vi "_MISC_ Cursor2Center.vi"(8 "Error In":errorcluster, 11 "WaveformGraph Ref":refnum<vi>) -> (0 "Error Out":errorcluster, 3 "XY":cluster{"X":dbl, "Y":dbl})   [LabVIEW 2014]
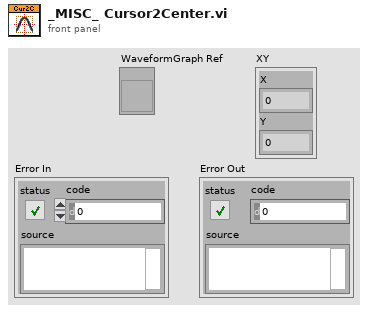
[diagram p1: front panel]
types:
  T1 = typedef "LVCursorListTypeDef.ctl" = cluster{"Name":string, "Color":u32, "Style":u8, "Point Style":u8, "Name Visible":bool, "Allow Drag":bool, "Cursor Mode":u32, "Plot":i32, "Index":i32, "Position":cluster{"X":dbl, "Y":dbl}, "X Scale":u32, "Y Scale":u32, "Watch Plots":i32[], "Watch All Plots":bool, "Plot Area":i32, "Label Offset":cluster{"X":dbl, "Y":dbl}}[]
  T2 = cluster{"Name":string, "Color":u32, "Style":u8, "Point Style":u8, "Name Visible":bool, "Allow Drag":bool, "Cursor Mode":u32, "Plot":i32, "Index":i32, "Position":cluster{"X":dbl, "Y":dbl}, "X Scale":u32, "Y Scale":u32, "Watch Plots":i32[], "Watch All Plots":bool, "Plot Area":i32, "Label Offset":cluster{"X":dbl, "Y":dbl}}
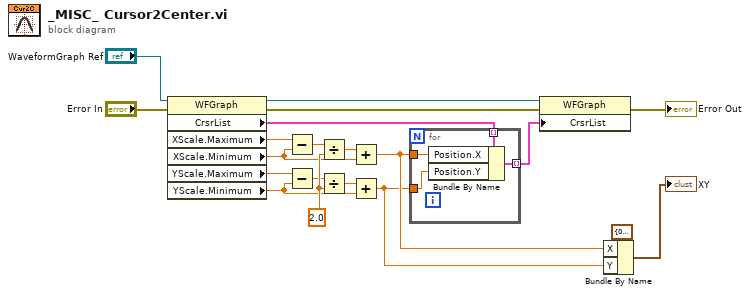
[diagram p0: block diagram]
diagram:
  w19 = 2.0 ("amplitude")
  n1 = property class="WFGraph"(reference="WaveformGraph Ref", error in="Error In") -> (reference out=w11:refnum<vi>, error out=w12:errorcluster, "CrsrList"=w20:T1, "XScale.Maximum"=w7:dbl, "XScale.Minimum"=w9:dbl, "YScale.Maximum"=w8:dbl, "YScale.Minimum"=w10:dbl)
  n2 = Subtract(x=w7, y=w9) -> (x-y=w16:dbl)
  n3 = Subtract(x=w8, y=w10) -> (x-y=w15:dbl)
  n4 = Divide(x=w16, y=w19) -> (x/y=w18:dbl)
  n5 = Divide(x=w15, y=w19) -> (x/y=w17:dbl)
  n6 = Add(x=w18, y=w9) -> (x+y=w2:dbl)
  n7 = Add(x=w17, y=w10) -> (x+y=w1:dbl)
  n8 = for {
    tunnel: w2 -> [w24]
    tunnel: w1 -> [w23]
    tunnel: [w22] -> w13 mode=indexing
    tunnel: w20 -> [w21] mode=indexing
    n9 = Bundle By Name(cluster=w21, "Position.X"=w24, "Position.Y"=w23) -> (w22:T2)
  }
  n10 = property class="WFGraph"(reference=w11, error in=w12, "CrsrList"=w13) -> (error out=→"Error Out":errorcluster)  [unwired: 1 out]
  n11 = Bundle By Name(cluster=cluster{"X":dbl, "Y":dbl} {"X"=0.0, "Y"=0.0} ("XY"), "X"=w2, "Y"=w1) -> (→"XY":cluster{"X":dbl, "Y":dbl})
